vi "Move Classes Out of Virtual Folder.vi"   [LabVIEW 2015]
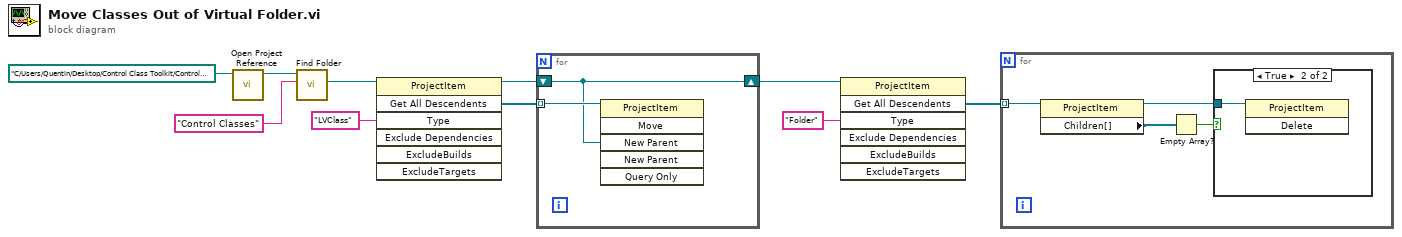
[diagram p0: block diagram]
diagram:
  n1 = call "Open Project Reference.vi"("Project Path"=path "C:/Users/Quentin/Desktop/Control Class Toolkit/Control Class Toolkit.lvproj") -> ("Project out"=w9:refnum<vi>)  [unwired: 10 in]
  n2 = call "Find Folder.vi"("Folder Name"="Control Classes", "Project in"=w9) -> ("Folder Refnum"=w7:refnum<vi>)  [unwired: 7 in, 2 out]
  n3 = invoke class="ProjectItem" method="Get All Descendents"(reference=w7, "Type"="LVClass") -> (reference out=w4:refnum<vi>, "All Descendents"=w5:refnum<vi>[])  [unwired: 5 in, 5 out]
  n4 = for {
    tunnel: w5 -> [w12] mode=indexing
    shift-right: [w11] -> w3
    shift-left: w4 -> [w11]
    n5 = invoke class="ProjectItem" method="Move"(reference=w12, "New Parent"=w11) -> ()  [unwired: 4 in, 6 out]
  }
  n6 = invoke class="ProjectItem" method="Get All Descendents"(reference=w3, "Type"="Folder") -> ("All Descendents"=w1:refnum<vi>[])  [unwired: 5 in, 6 out]
  n7 = for {
    tunnel: w1 -> [w16] mode=indexing
    n8 = property class="ProjectItem"(reference=w16) -> (reference out=w13:refnum<vi>, "Children[]"=w15:refnum<vi>[])  [unwired: 1 in, 1 out]
    n9 = Empty Array?(array=w15) -> (empty?=w14:bool)
    n10 = case shown="True" w14 {
      tunnel: w13 -> [_ w17]
      frame False {
      }
      frame True {
        n11 = invoke class="ProjectItem" method="Delete"(reference=w17) -> ()  [unwired: 2 in, 3 out]
      }
    }
  }
